vi "Get ConfigChangedEvent.vi"(8 "error in (no error)":errorcluster, 11 "Attribute.Config in":refnum<class "Attribute.Config.lvclass">) -> (0 "error out":errorcluster, 2 "Config change event":refnum<user-event>, 3 "Attribute.Config out":refnum<class "Attribute.Config.lvclass">)   [LabVIEW 2019, in "Attribute.Config.lvclass"]
doc: "JKI State Machine Objects (SMO) 1.3.0.56\nJKI - JKI\nCopyright (c) 2017, JKI"
uses:
  Attribute.Config.lvclass
  Attribute.Config.lvclass/Attribute.Config.ctl
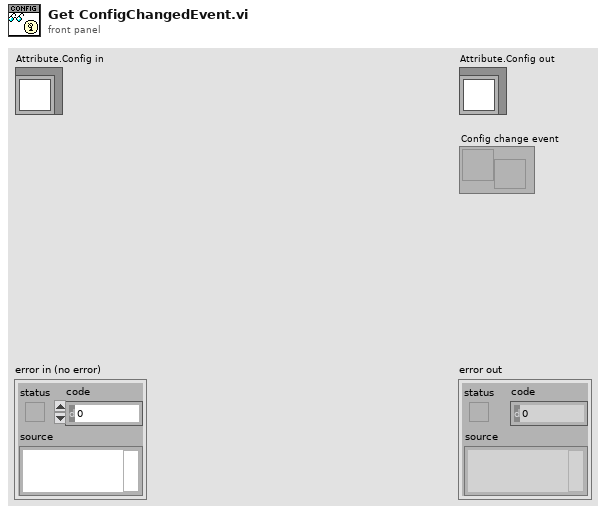
[diagram p1: front panel]
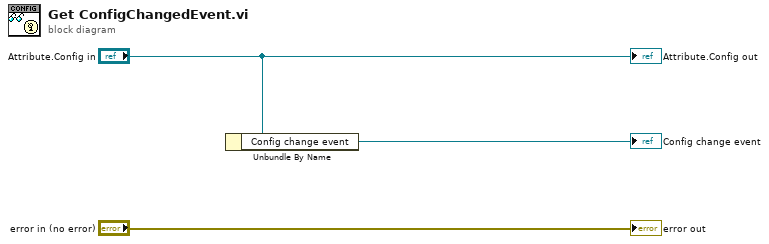
[diagram p0: block diagram]
diagram:
  n1 = Unbundle By Name("Attribute.Config in") -> ("Config change event"=→"Config change event":refnum<user-event>)
  "error out" <- "error in (no error)"
  "Attribute.Config out" <- "Attribute.Config in"
